vi "General Linear Fit.vi"(0 "Y":dbl[](array[numeric]), 1 "covariance selector":T4(ring), 5 "H":dbl[][](array[numeric]), 7 "Weight":dbl[](array[numeric]), 9 "tolerance":dbl=0.0001, 11 "method":T1 items=["Least Square", "Least Absolute Residual", "Bisquare"], 13 "algorithm":T3 items=["SVD", "Givens", "Givens2", "Householder", "LU Decomposition", "Cholesky", "SVD for Rank Deficient H"]) -> (4 "Best Fit":dbl[](array[numeric]), 6 "Coefficients":dbl[](array[numeric]), 8 "Covariance":T2, 10 "Weight Out":dbl[](array[numeric]), 14 "residue":dbl, 15 "error":i32)   [LabVIEW 2024, in "NI_AALPro.lvlib"]
doc: "<p>Finds the <em>k</em>-dimension linear curve values and the set of <em>k</em>-dimension linear fit coefficients, which describe the <em>k</em>-dimension linear curve that best represents the input data set using the Least Square, Least Absolute Residual, or Bisquare method.</p>"
uses:
  NI_AALPro.lvlib
  General Linear Fit Algorithm.ctl
  RealMatrix.ctl
  Curve Fitting Criteria.ctl
  Array To Matrix.vi
  Array To Matrix - RA2.vi
  NI_Matrix.lvlib
panel:
  # "General Linear Fit"
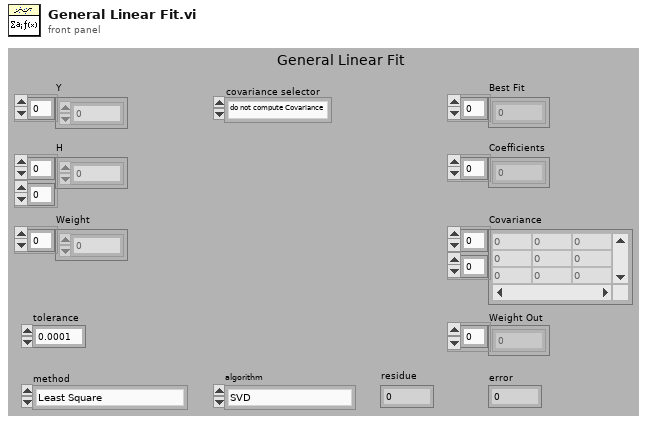
[diagram p1: front panel]
types:
  T1 = typedef "NI_AALPro.lvlib/Curve Fitting Criteria.ctl" = u16
  T2 = typedef "NI_Matrix.lvlib/RealMatrix.ctl" = dbl[][]
  T3 = typedef "NI_AALPro.lvlib/General Linear Fit Algorithm.ctl" = u16
  T4 = enum32{"do not compute Covariance", " compute Covariance"}
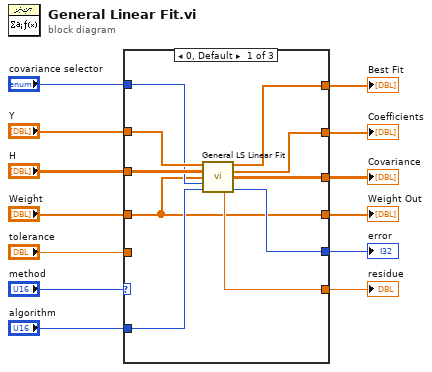
[diagram p0: block diagram]
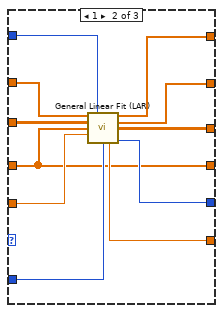
[diagram p2: hidden frame]
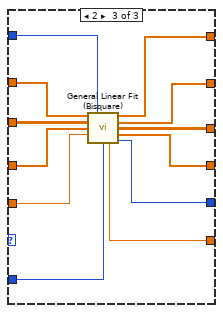
[diagram p3: hidden frame]
diagram:
  n1 = case shown="0, Default" "method" {
    tunnel: "H" -> [w23 w34 w46]
    tunnel: "Y" -> [w22 w33 w45]
    tunnel: "Weight" -> [w14 w24 w44]
    tunnel: "covariance selector" -> [w15 w25 w36]
    tunnel: "algorithm" -> [w16 w26 w37]
    tunnel: [w21 w32 w43] -> w7
    tunnel: [w20 w31 w42] -> w6
    tunnel: [w19 w30 w41] -> w5
    tunnel: [w18 w29 w40] -> w4
    tunnel: [w17 w28 w39] -> w3
    tunnel: "tolerance" -> [_ w27 w38]
    tunnel: [w14 w24 w35] -> w1
    frame 0, Default {
      n2 = call "General LS Linear Fit.vi"("Y"=w22, "H"=w23, "Weight"=w14, "covariance selector"=w15, "algorithm"=w16) -> ("Best Fit"=w21:dbl[], "Coefficients"=w20:dbl[], "Covariance"=w19:T2, "mse"=w17:dbl, "error"=w18:i32)  [unwired: 6 out]
    }
    frame 1 {
      n3 = call "General Linear Fit (LAR).vi"("Y"=w33, "covariance selector"=w25, "H"=w34, "Weight"=w24, "tolerance"=w27, "algorithm"=w26) -> ("Best Fit"=w32:dbl[], "Coefficients"=w31:dbl[], "Covariance"=w30:T2, "residue"=w28:dbl, "error"=w29:i32)  [unwired: 1 in, 4 out]
    }
    frame 2 {
      n4 = call "General Linear Fit (Bisquare).vi"("Y"=w45, "covariance selector"=w36, "H"=w46, "Weight"=w44, "tolerance"=w38, "algorithm"=w37) -> ("Best Fit"=w43:dbl[], "Coefficients"=w42:dbl[], "Covariance"=w41:T2, "Weight Out"=w35:dbl[], "residue"=w39:dbl, "error"=w40:i32)  [unwired: 1 in, 3 out]
    }
  }
  "Best Fit" <- w7
  "Coefficients" <- w6
  "Covariance" <- w5
  "residue" <- w3
  "error" <- w4
  "Weight Out" <- w1
